vi "Main.vi"(11 "Module Number":dbl=1.0) -> ()   [LabVIEW 2015, in "Copy of Untitled Library 1.lvlib"]
uses:
  Copy of Untitled Library 1.lvlib
  Controls/Control 1.ctl
  <vilib>/Utility/miscctls.llb/LVPointTypeDef.ctl
  Controls/Enum Constant.ctl
  <userlib>/origin_lib_main/ui_msg_lib/CTRL/Display MSG Types.ctl
  <userlib>/origin_lib_main/ui_msg_lib/MSG Library.lvlib
  <userlib>/origin_lib_main/virtual_keyboard_lib/virtual_keyboard.lvlib
panel:
  out "Primery key values":string[](array[string])
  out "subarray":string[](array[string])
  in  "Tab Control":enum32{"Page 1", "Page 2"}(tab)
  in  "close button":bool
  in  "Close Batch":bool
  in  "Open Batch":bool
  in  "New Product":bool
  in  "Delete Product":bool
  in  "Reset Button":bool
  in  "Edit Button":bool
  in  "Delete Batch":bool
  in  "ADD Batch":bool
  in  "Logo 4":bool
  in  "Page Header 2":string="                                                                           BATCH PAGE"
  in  "Check Batch Status":bool caption="Open"
  in  "Batch Data 3":T1 caption="Batch Data"
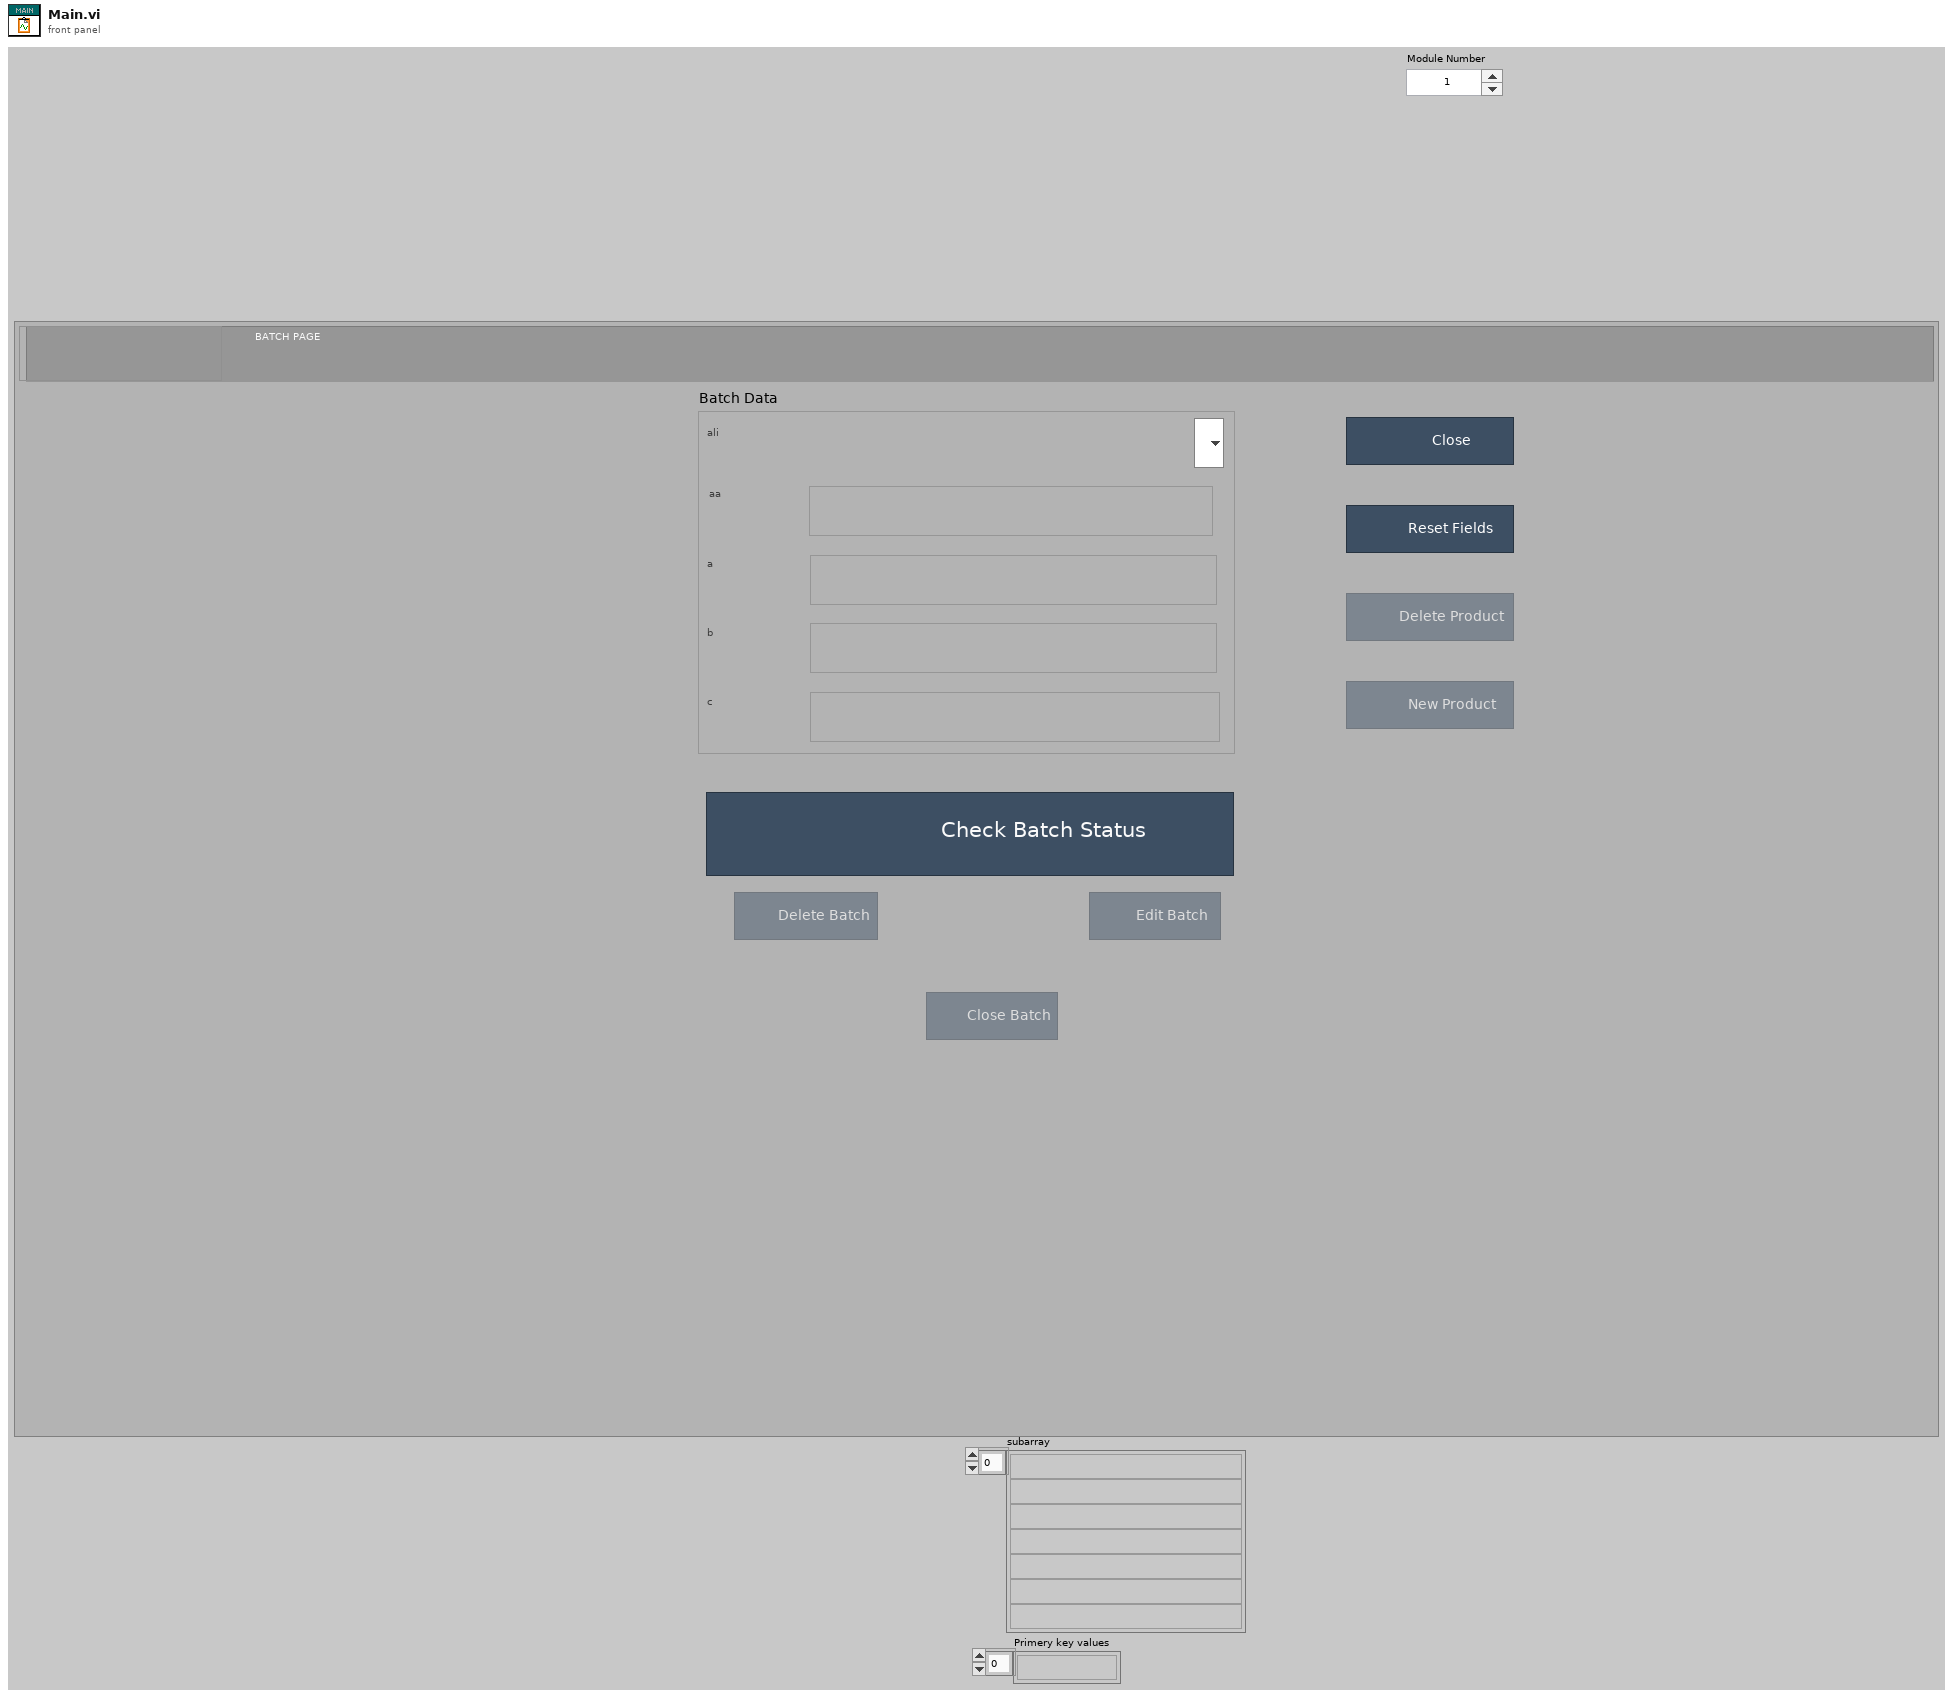
[diagram p1: front panel]
types:
  T1 = typedef "Copy of Untitled Library 1.lvlib/Control 1.ctl" = cluster{"DATA":string, "DATA 2":string, "DATA 3":string, "DATA 4":string, "DATA 5":string, "DATA 6":string, "DATA 7":string, "DATA 8":string, "DATA 9":string, "DATA 10":string, "Product":string}
  T2 = typedef "LVPointTypeDef.ctl" = cluster{"Horizontal":i16, "Vertical":i16}
  T3 = enum32{"Invalid", "Standard", "Closed", "Hidden", "Minimized", "Maximized"}
  T4 = typedef "Enum Constant.ctl" = enum16{"Init", "Read", "Write"}
  T5 = enum8{"Enabled", "Disabled", "Disabled and Grayed Out"}
  T6 = typedef "MSG Library.lvlib/Display MSG Types.ctl" = enum16{"Display MSG 1", "Display MSG 2", "Display MSG Load", "End MSG Load ", "Display 2 STR MSG"}
  T7 = typedef "FGV Data.ctl" = T8[]
  T8 = typedef "FGV Cluster Data.ctl" = cluster{"Manual/Automatic":bool, "UI Controllers ":string[], "UI Primery Key ":dbl[], "Caller Queue & MSG":T9, "Module ID":dbl, "DB Reference In":T10, "Products Columns":string[], "Cluster":cluster{"Delete Product":enum8{"Enabled", "Disabled", "Disabled and Grayed Out"}, "Add Product ":enum8{"Enabled", "Disabled", "Disabled and Grayed Out"}, "EDIT BATCH":enum8{"Enabled", "Disabled", "Disabled and Grayed Out"}, "Open Batch ":enum8{"Enabled", "Disabled", "Disabled and Grayed Out"}, "Close Batch":enum8{"Enabled", "Disabled", "Disabled and Grayed Out"}, "Delete Batch":enum8{"Enabled", "Disabled", "Disabled and Grayed Out"}, "Add Batch ":enum8{"Enabled", "Disabled", "Disabled and Grayed Out"}}}
  T9 = typedef "Queue and Caller MSG.ctl" = cluster{"Caller Queue":refnum<queue>, "Caller MSG":string}
  T10 = typedef "NI_Database_API.lvlib/Conn ObjectReference.ctl" = refnum<k1>
  T11 = cluster{"Delete Product":enum8{"Enabled", "Disabled", "Disabled and Grayed Out"}, "Add Product ":enum8{"Enabled", "Disabled", "Disabled and Grayed Out"}, "EDIT BATCH":enum8{"Enabled", "Disabled", "Disabled and Grayed Out"}, "Open Batch ":enum8{"Enabled", "Disabled", "Disabled and Grayed Out"}, "Close Batch":enum8{"Enabled", "Disabled", "Disabled and Grayed Out"}, "Delete Batch":enum8{"Enabled", "Disabled", "Disabled and Grayed Out"}, "Add Batch ":enum8{"Enabled", "Disabled", "Disabled and Grayed Out"}}
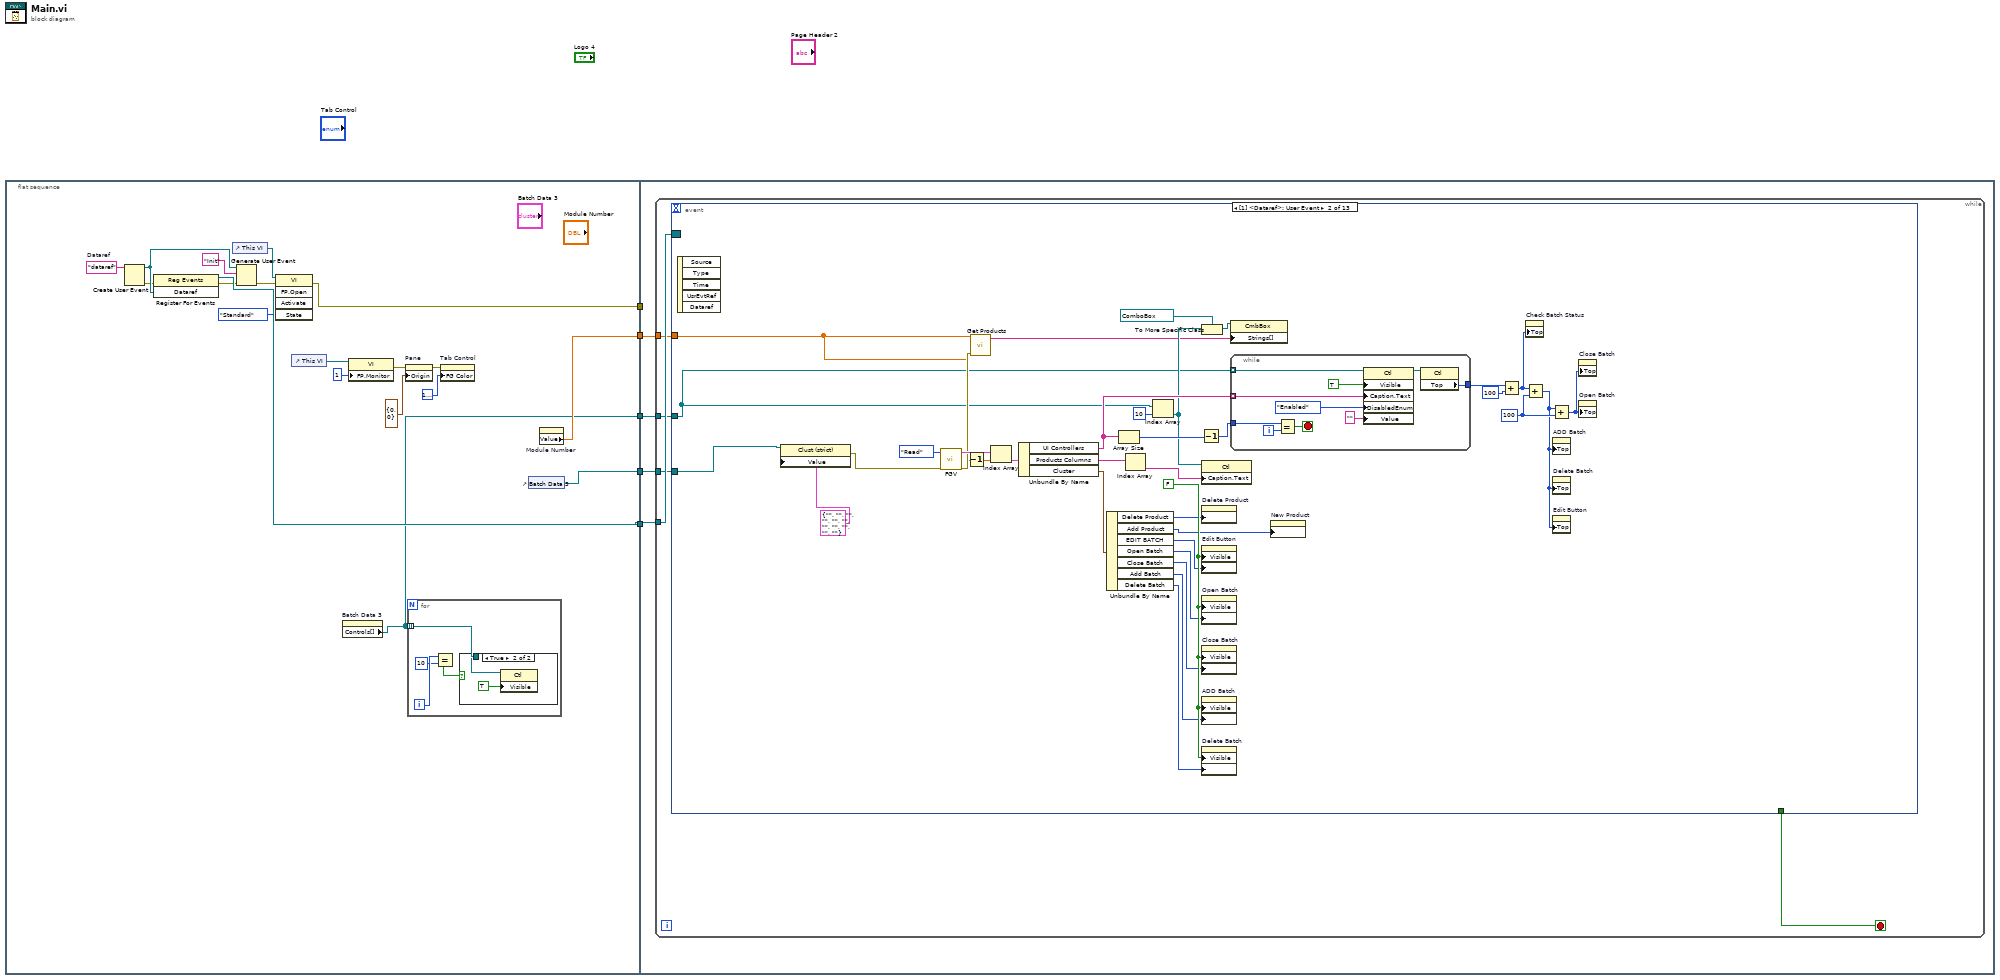
[diagram p0: block diagram]
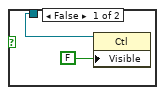
[diagram p2: hidden frame]
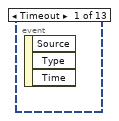
[diagram p3: hidden frame]
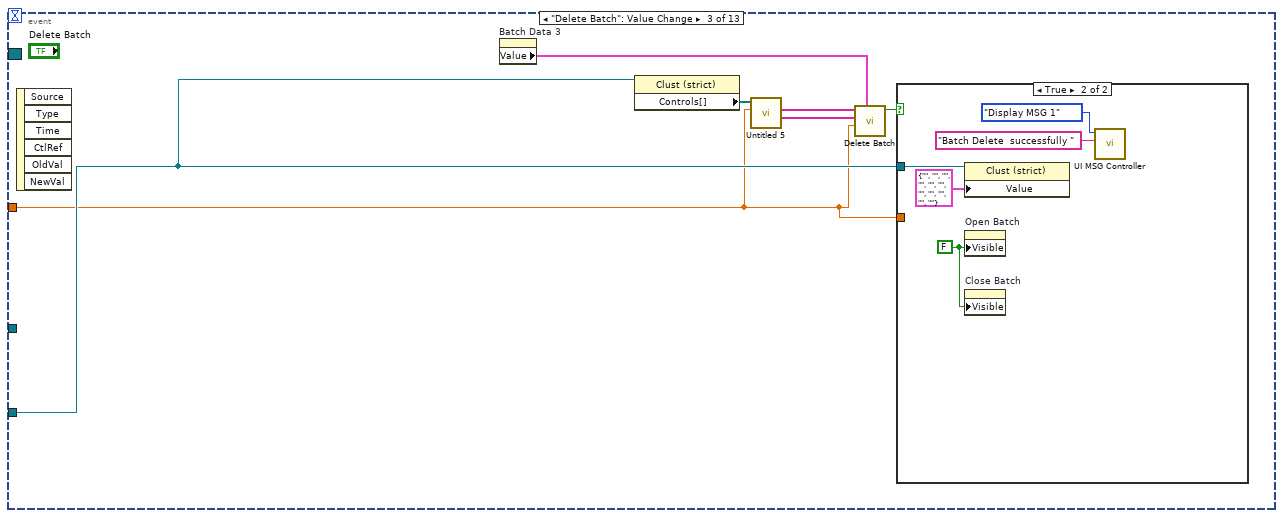
[diagram p4: hidden frame]
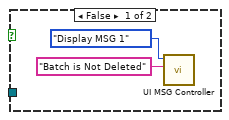
[diagram p5: hidden frame]
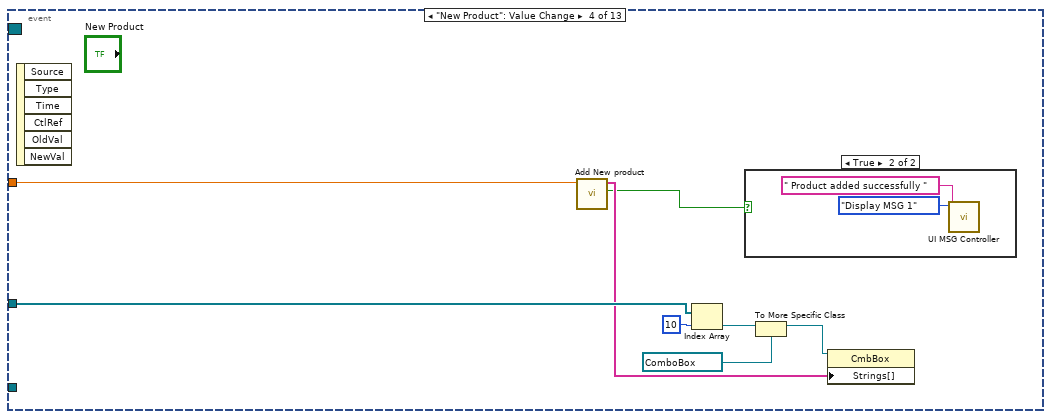
[diagram p6: hidden frame]
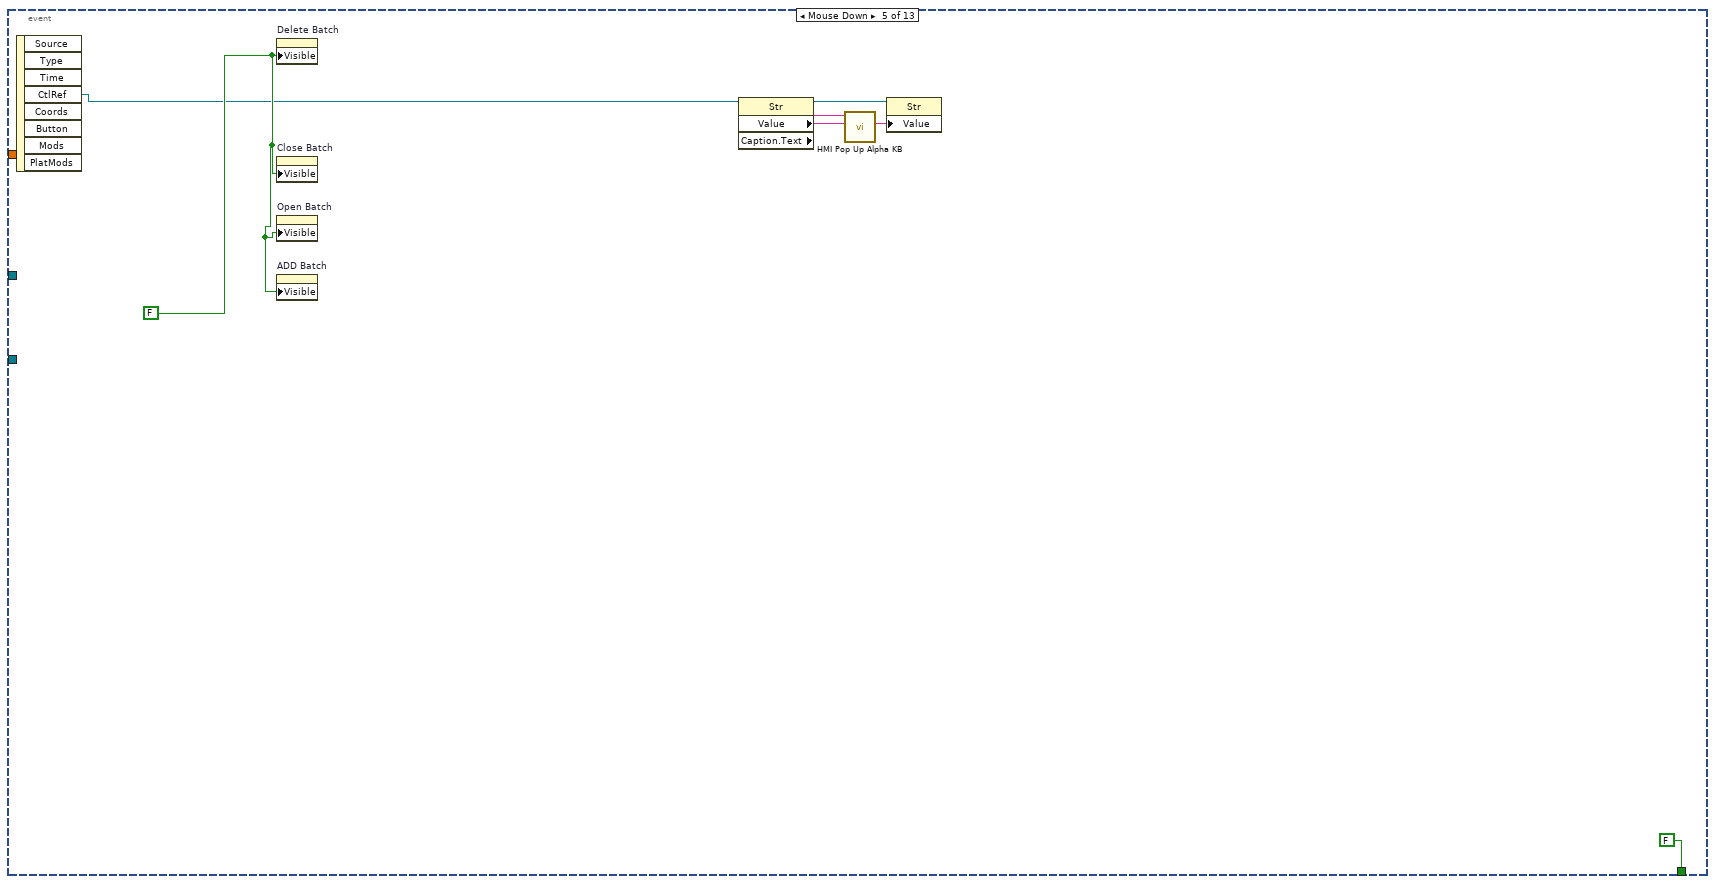
[diagram p8: hidden frame]
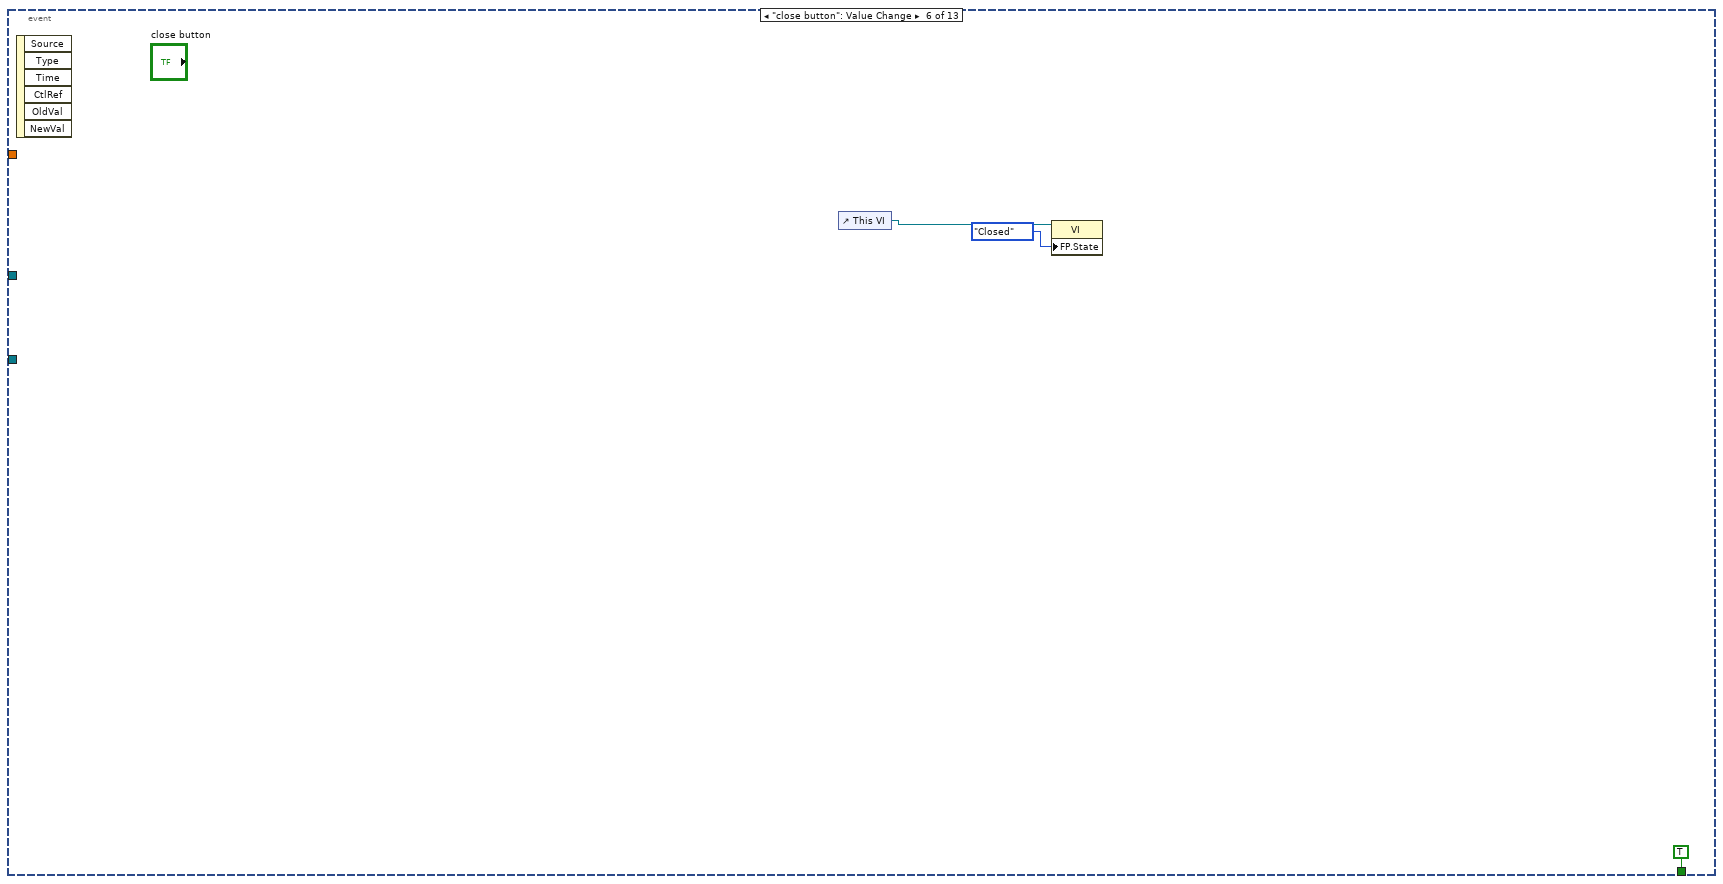
[diagram p9: hidden frame]
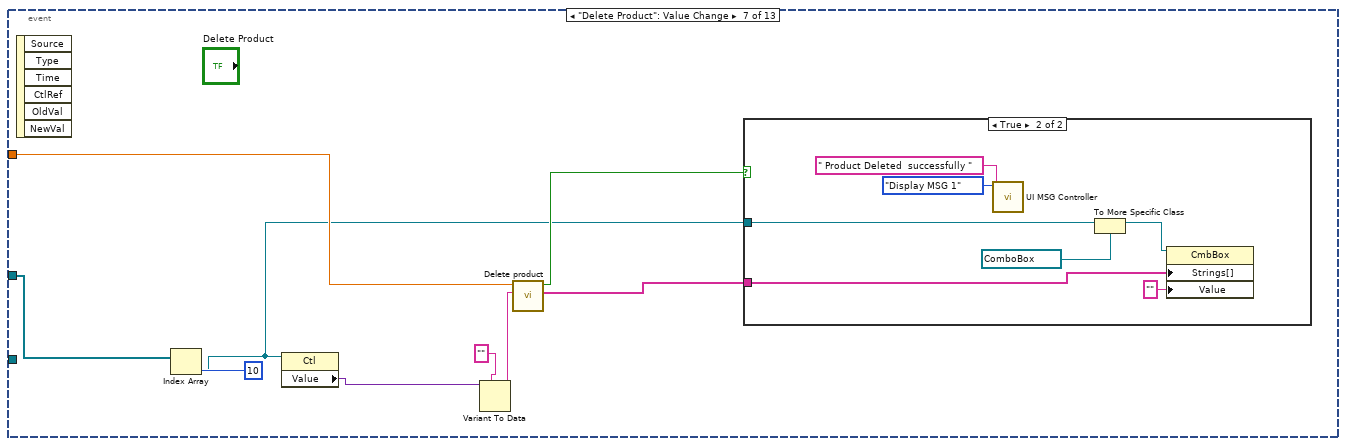
[diagram p10: hidden frame]
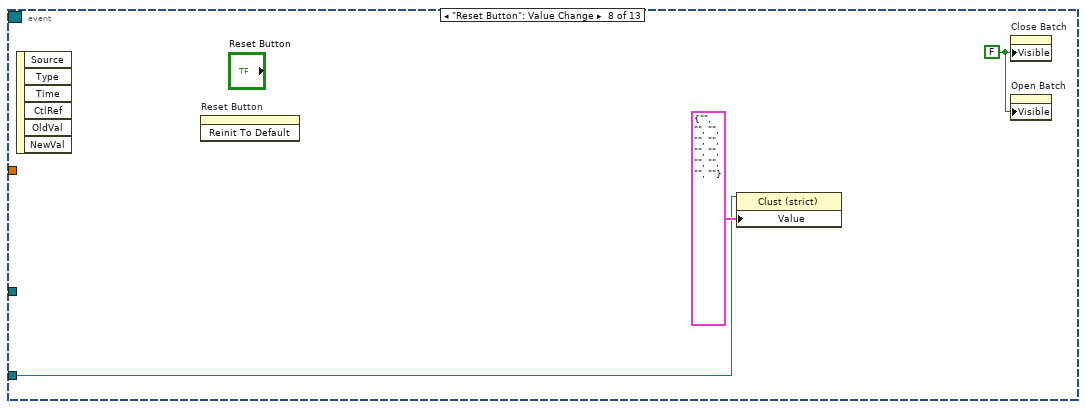
[diagram p12: hidden frame]
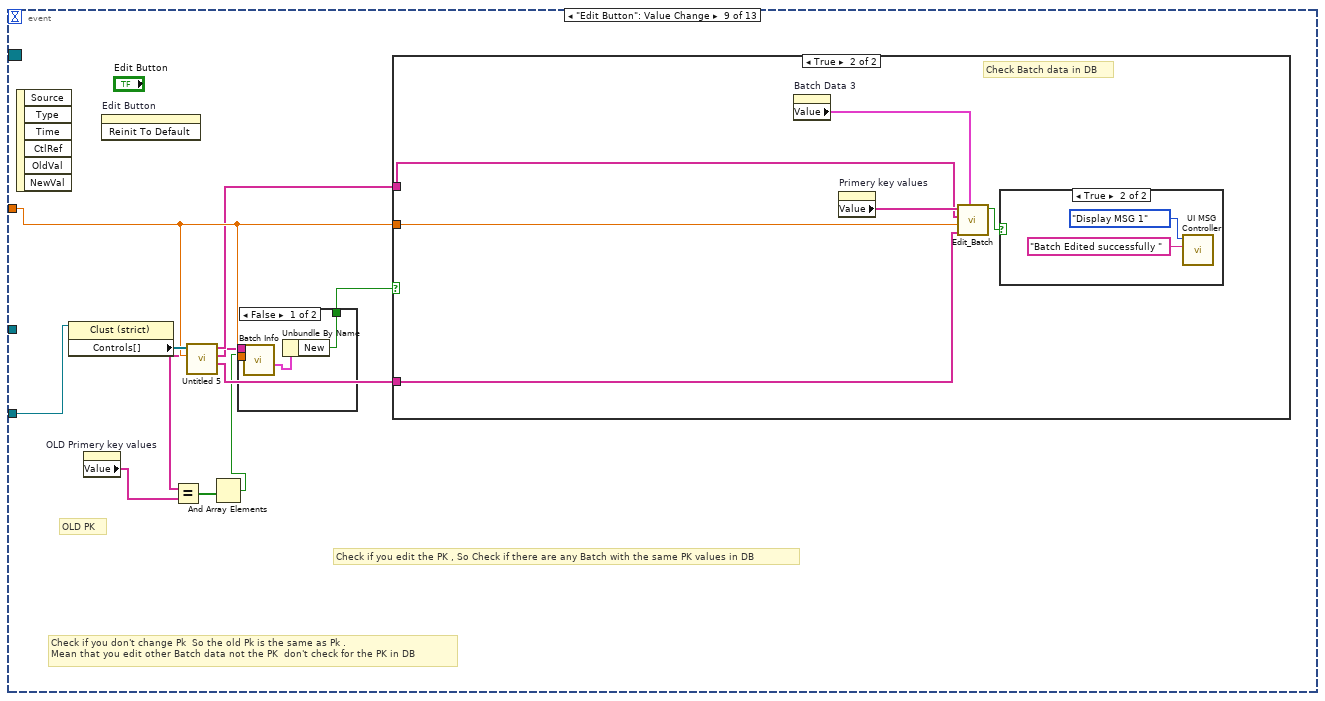
[diagram p13: hidden frame]
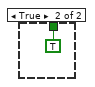
[diagram p14: hidden frame]
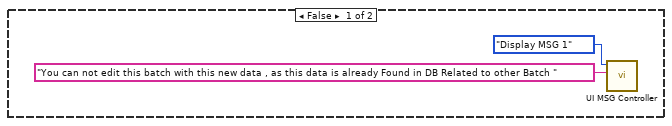
[diagram p15: hidden frame]
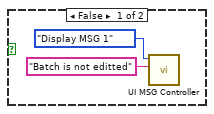
[diagram p16: hidden frame]
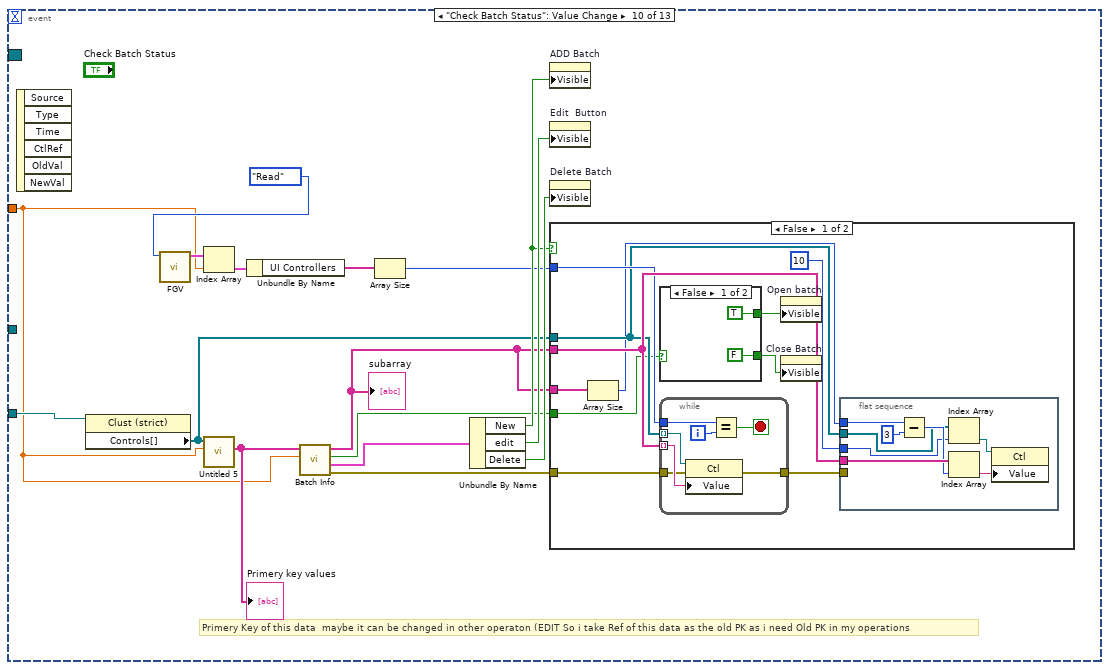
[diagram p17: hidden frame]
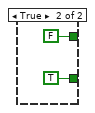
[diagram p18: hidden frame]
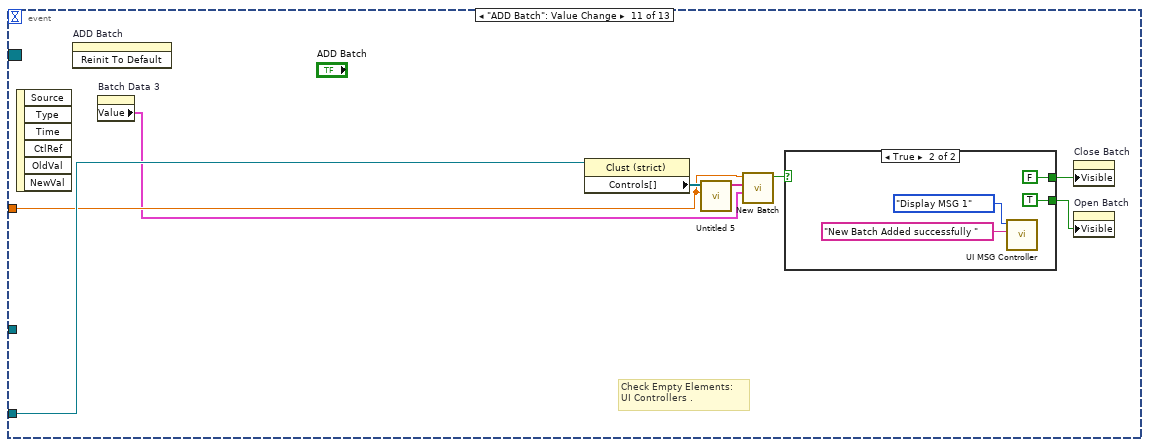
[diagram p20: hidden frame]
diagram:
  n1 = flat-sequence {
    tunnel: [w21] -> w5
    tunnel: [w15] -> w4
    tunnel: [w8] -> w3
    tunnel: [w7] -> w2
    tunnel: [w6] -> w1
    tunnel: w5 -> [w36]
    tunnel: w4 -> [_]
    tunnel: w3 -> [w35]
    tunnel: w2 -> [w34]
    tunnel: w1 -> [w33]
    frame #0 {
      w24 = "dataref"  # Dataref
      n2 = Create User Event(user event datatype=w24) -> (user event=w22:refnum<user-event>, error out=w19:errorcluster)  [unwired: 1 in]
      n3 = register-events(error in=w19, w22) -> (reference out=w21:refnum<event-registration>, error out=w20:errorcluster)  [unwired: 1 in]
      n4 = control-ref of="This VI"() -> (w18:refnum<vi>)
      n5 = Generate User Event(user event=w22, event data cluster="Init" ("event data"), error in=w20) -> (error out=w16:errorcluster)  [unwired: 1 in, 1 out]
      n6 = invoke class="VI" method="FP.Open"(reference=w18, error in=w16, "State"=T3."Standard") -> (error out=w15:errorcluster)  [unwired: 2 in, 4 out]
      n7 = control-ref of="This VI"() -> (w14:refnum<vi>)
      n8 = property on="Batch Data 3" class="Clust (strict)"() -> ("Controls[]"=w7:refnum<vi>[])  [unwired: 2 in, 2 out]
      n9 = property class="VI"(reference=w14, "FP.Monitor"=u16 1 ("Front Panel Window:Monitor")) -> (error out=w11:errorcluster)  [unwired: 1 in, 1 out]
      n10 = property on="Pane" class="Pane"(error in=w11, "Origin"=T2 {"Horizontal"=0, "Vertical"=0}) -> (error out=w9:errorcluster)  [unwired: 1 in, 1 out]
      n11 = for {
        tunnel: w7 -> [w28] mode=indexing
        i -> [w27]
        n12 = Equal?(x=w27, y=10) -> (x = y?=w25:bool)
        n13 = case shown="True" w25 {
          tunnel: w28 -> [w29 w31]
          frame False {
            n14 = property class="Ctl"(reference=w29, "Visible"=FALSE) -> ()  [unwired: 1 in, 2 out]
          }
          frame True {
            n15 = property class="Ctl"(reference=w31, "Visible"=TRUE) -> ()  [unwired: 1 in, 2 out]
          }
        }
      }
      n16 = property on="Tab Control" class="TabCtl (strict)"(error in=w9, "FG Color"=u32 16777225) -> ()  [unwired: 1 in, 2 out]
      n17 = control-ref of="Batch Data 3"() -> (w6:refnum<vi>)
      n18 = property on="Module Number" class="DigNum (strict)"() -> ("Value"=w8:dbl)  [unwired: 2 in, 2 out]
    }
    frame #1 {
      n19 = while {
        tunnel: w36 -> [w41]
        tunnel: w35 -> [w40]
        tunnel: w34 -> [w39]
        tunnel: w33 -> [w38]
        stop <- w37 stop-if-true
        n20 = event shown="[1] <Dataref>: User Event" {
          selector: w41 -> [_ _ _ _ _ _ _ _ _ _ _ _ _]
          dyn-events: _ -> [_ _ _ _ _ _ _ _ _ _ _ _ _]
          timeout: _ -> [_ _ _ _ _ _ _ _ _ _ _ _ _]
          tunnel: w40 -> [_ w50 w88 w108 _ _ w129 _ w147 w169 w214 w230 w250]
          tunnel: w39 -> [_ w52 _ w103 _ _ w128 _ _ _ _ _ _]
          tunnel: w38 -> [_ w51 w89 _ _ _ _ w137 w146 w173 w215 w229 w249]
          tunnel: [_ _ _ _ FALSE TRUE _ _ _ _ _ _ _] -> w37
          event Timeout {
            n21 = event-data() -> ()  [unwired: 1 in, 3 out]
          }
          event User Event {
            w66 = 100 ("y")
            w67 = FALSE ("Visible")
            n22 = event-data() -> ()  [unwired: 1 in, 5 out]
            n23 = property class="Clust (strict)"(reference=w51, "Value"=T1 {"DATA"="", "DATA 2"="", "DATA 3"="", "DATA 4"="", "DATA 5"="", "DATA 6"="", "DATA 7"="", "DATA 8"="", "DATA 9"="", "DATA 10"="", "Product"=""}) -> (error out=w53:errorcluster)  [unwired: 1 in, 1 out]
            n24 = call "FGV.vi"("error out 2"=w53, "Enum"=Enum_Constant."Read") -> ("error out"=w60:errorcluster, "Read Data"=w75:T7)  [unwired: 8 in]
            n25 = Decrement(x=w50) -> (x-1=w55:dbl)
            n26 = call "Get Products.vi"("error in (no error) 5"=w60, "Module Number  2"=w50) -> ("subarray"=w56:string[])  [unwired: 8 in, 1 out]
            n27 = Index Array(array=w75, index=w55) -> (element=w74:T8)
            n28 = Unbundle By Name(w74) -> ("UI Controllers"=w73:string[], "Products Columns"=w62:string[], "Cluster"=w49:T11)
            n29 = Unbundle By Name(w49) -> ("Delete Product"=w48:T5, "Add Product"=w47:T5, "EDIT BATCH"=w46:T5, "Open Batch"=w45:T5, "Close Batch"=w44:T5, "Add Batch"=w43:T5, "Delete Batch"=w42:T5)
            n30 = Array Size(array=w73) -> (size(s)=w70:i32)
            n31 = Index Array(array=w62) -> (element=w61:string)  [unwired: 1 in]
            n32 = Index Array(array=w52, index=10) -> (element=w57:refnum<vi>)
            n33 = Decrement(x=w70) -> (x-1=w69:i32)
            n34 = To More Specific Class(target class=refnum<vi> refnum ("Product"), reference=w57) -> (specific class reference=w59:refnum<vi>)  [unwired: 1 in, 1 out]
            n35 = property class="Ctl"(reference=w57, "Caption.Text"=w61) -> ()  [unwired: 1 in, 2 out]
            n36 = property on="Delete Product" class="Bool"("DisabledEnum"=w48) -> ()  [unwired: 2 in, 2 out]
            n37 = property on="Edit Button" class="Bool"("Visible"=w67, "DisabledEnum"=w46) -> ()  [unwired: 2 in, 2 out]
            n38 = property on="Open Batch" class="Bool"("Visible"=w67, "DisabledEnum"=w45) -> ()  [unwired: 2 in, 2 out]
            n39 = property on="Close Batch" class="Bool"("Visible"=w67, "DisabledEnum"=w44) -> ()  [unwired: 2 in, 2 out]
            n40 = property on="ADD Batch" class="Bool (strict)"("Visible"=w67, "DisabledEnum"=w43) -> ()  [unwired: 2 in, 2 out]
            n41 = property on="Delete Batch" class="Bool"("Visible"=w67, "DisabledEnum"=w42) -> ()  [unwired: 2 in, 2 out]
            n42 = property class="CmbBox"(reference=w59, "Strings[]"=w56) -> ()  [unwired: 1 in, 2 out]
            n43 = while {
              tunnel: w73 -> [w82] mode=indexing
              tunnel: w69 -> [w86]
              tunnel: [w80] -> w71
              tunnel: w52 -> [w79] mode=indexing
              i -> [w85]
              stop <- w84 stop-if-true
              n44 = Equal?(x=w86, y=w85) -> (x = y?=w84:bool)
              n45 = property class="Ctl"(reference=w79, "Visible"=TRUE, "Caption.Text"=w82, "DisabledEnum"=T5."Enabled" ("Disabled"), "Value"="" ("String")) -> (reference out=w81:refnum<vi>)  [unwired: 1 in, 1 out]
              n46 = property class="Ctl"(reference=w81) -> ("Top"=w80:i32)  [unwired: 1 in, 2 out]
            }
            n47 = property on="New Product" class="Bool"("DisabledEnum"=w47) -> ()  [unwired: 2 in, 2 out]
            n48 = Add(x=w71, y=100) -> (x+y=w68:i32)
            n49 = Add(x=w68, y=w66) -> (x+y=w65:i32)
            n50 = property on="Check Batch Status" class="Bool"("Top"=w68) -> ()  [unwired: 2 in, 2 out]
            n51 = Add(x=w65, y=w66) -> (x+y=w64:i32)
            n52 = property on="ADD Batch" class="Bool (strict)"("Top"=w65) -> ()  [unwired: 2 in, 2 out]
            n53 = property on="Delete Batch" class="Bool"("Top"=w65) -> ()  [unwired: 2 in, 2 out]
            n54 = property on="Edit Button" class="Bool"("Top"=w65) -> ()  [unwired: 2 in, 2 out]
            n55 = property on="Close Batch" class="Bool"("Top"=w64) -> ()  [unwired: 2 in, 2 out]
            n56 = property on="Open Batch" class="Bool"("Top"=w64) -> ()  [unwired: 2 in, 2 out]
          }
          event "Delete Batch": Value Change {
            n57 = event-data() -> ()  [unwired: 1 in, 6 out]
            n58 = property on="Batch Data 3" class="Clust (strict)"() -> ("Value"=w87:T1)  [unwired: 2 in, 2 out]
            n59 = property class="Clust (strict)"(reference=w89) -> ("Controls[]"=w93:refnum<vi>[])  [unwired: 1 in, 2 out]
            n60 = call "Untitled 5.vi"("Module Number"=w88, "Controls[]"=w93) -> ("Primery key Names"=w91:string[], "Primery key values"=w92:string[])  [unwired: 7 in, 1 out]
            n61 = call "Delete Batch .vi"("Batch Data 3"=w87, "Module Number"=w88, "Primery key names"=w91, "Primery key last values"=w92) -> ("Sucess ?"=w90:bool)  [unwired: 7 in]
            n62 = case shown="True" w90 {
              tunnel: w89 -> [_ w98]
              tunnel: w88 -> [_ _]
              frame False {
                n63 = call <userlib>:"UI MSG Controller.vi"("MSG"="Batch is Not Deleted", "Display MSG Type"=Display_MSG_Types."Display MSG 1") -> ()  [unwired: 6 in, 4 out]
              }
              frame True {
                w96 = FALSE ("Visible")
                n64 = property class="Clust (strict)"(reference=w98, "Value"=T1 {"DATA"="", "DATA 2"="", "DATA 3"="", "DATA 4"="", "DATA 5"="", "DATA 6"="", "DATA 7"="", "DATA 8"="", "DATA 9"="", "DATA 10"="", "Product"=""}) -> ()  [unwired: 1 in, 2 out]
                n65 = property on="Open Batch" class="Bool"("Visible"=w96) -> ()  [unwired: 2 in, 2 out]
                n66 = property on="Close Batch" class="Bool"("Visible"=w96) -> ()  [unwired: 2 in, 2 out]
                n67 = call <userlib>:"UI MSG Controller.vi"("MSG"="Batch Delete  successfully ", "Display MSG Type"=Display_MSG_Types."Display MSG 1") -> ()  [unwired: 6 in, 4 out]
              }
            }
          }
          event "New Product": Value Change {
            n68 = event-data() -> ()  [unwired: 1 in, 6 out]
            n69 = call "Add New product.vi"("Module Number  2"=w108) -> ("Sucess ?"=w101:bool, "subarray"=w102:string[])  [unwired: 8 in, 1 out]
            n70 = Index Array(array=w103, index=10) -> (element=w104:refnum<vi>)
            n71 = case shown="True" w101 {
              frame False {
              }
              frame True {
                n72 = call <userlib>:"UI MSG Controller.vi"("MSG"=" Product added successfully ", "Display MSG Type"=Display_MSG_Types."Display MSG 1") -> ()  [unwired: 6 in, 4 out]
              }
            }
            n73 = To More Specific Class(target class=refnum<vi> refnum ("Product"), reference=w104) -> (specific class reference=w106:refnum<vi>)  [unwired: 1 in, 1 out]
            n74 = property class="CmbBox"(reference=w106, "Strings[]"=w102) -> ()  [unwired: 1 in, 2 out]
          }
          event Mouse Down {
            w117 = FALSE ("Visible")
            n75 = event-data() -> ("CtlRef"=w112:refnum<vi>)  [unwired: 1 in, 7 out]
            n76 = property on="Delete Batch" class="Bool"("Visible"=w117) -> ()  [unwired: 2 in, 2 out]
            n77 = property on="Close Batch" class="Bool"("Visible"=w117) -> ()  [unwired: 2 in, 2 out]
            n78 = property on="Open Batch" class="Bool"("Visible"=w117) -> ()  [unwired: 2 in, 2 out]
            n79 = property on="ADD Batch" class="Bool (strict)"("Visible"=w117) -> ()  [unwired: 2 in, 2 out]
            n80 = property class="Str"(reference=w112) -> (reference out=w114:refnum<vi>, "Value"=w116:string, "Caption.Text"=w113:string)  [unwired: 1 in, 1 out]
            n81 = call <userlib>:"HMI Pop Up Alpha KB.vi"("String In"=w116, "Message In"=w113) -> ("String Out"=w115:string)  [unwired: 7 in, 2 out]
            n82 = property class="Str"(reference=w114, "Value"=w115) -> ()  [unwired: 1 in, 2 out]
          }
          event "close button": Value Change {
            n83 = event-data() -> ()  [unwired: 1 in, 6 out]
            n84 = control-ref of="This VI"() -> (w120:refnum<vi>)
            n85 = property class="VI"(reference=w120, "FP.State"=T3."Closed" ("Front Panel Window:State")) -> ()  [unwired: 1 in, 2 out]
          }
          event "Delete Product": Value Change {
            n86 = event-data() -> ()  [unwired: 1 in, 6 out]
            n87 = Index Array(array=w128, index=10) -> (element=w121:refnum<vi>)
            n88 = property class="Ctl"(reference=w121) -> ("Value"=w126:variant)  [unwired: 1 in, 2 out]
            n89 = Variant To Data(type="", Variant=w126) -> (data=w124:string)  [unwired: 1 in, 1 out]
            n90 = call "Delete product.vi"("String"=w124, "Module Number  2"=w129) -> ("subarray"=w122:string[], "Sucess ?"=w123:bool)  [unwired: 7 in, 1 out]
            n91 = case shown="True" w123 {
              tunnel: w122 -> [_ w132]
              tunnel: w121 -> [_ w131]
              frame False {
              }
              frame True {
                n92 = call <userlib>:"UI MSG Controller.vi"("MSG"=" Product Deleted  successfully ", "Display MSG Type"=Display_MSG_Types."Display MSG 1") -> ()  [unwired: 6 in, 4 out]
                n93 = To More Specific Class(target class=refnum<vi> refnum ("Product"), reference=w131) -> (specific class reference=w133:refnum<vi>)  [unwired: 1 in, 1 out]
                n94 = property class="CmbBox"(reference=w133, "Strings[]"=w132, "Value"="") -> ()  [unwired: 1 in, 2 out]
              }
            }
          }
          event "Reset Button": Value Change {
            w138 = FALSE ("Visible")
            n95 = event-data() -> ()  [unwired: 1 in, 6 out]
            n96 = invoke on="Reset Button" class="Bool" method="Reinit To Default"() -> ()  [unwired: 3 in, 3 out]
            n97 = property class="Clust (strict)"(reference=w137, "Value"=T1 {"DATA"="", "DATA 2"="", "DATA 3"="", "DATA 4"="", "DATA 5"="", "DATA 6"="", "DATA 7"="", "DATA 8"="", "DATA 9"="", "DATA 10"="", "Product"=""}) -> ()  [unwired: 1 in, 2 out]
            n98 = property on="Close Batch" class="Bool"("Visible"=w138) -> ()  [unwired: 2 in, 2 out]
            n99 = property on="Open Batch" class="Bool"("Visible"=w138) -> ()  [unwired: 2 in, 2 out]
          }
          event "Edit Button": Value Change {
            # "Check if you don't change Pk  So the old Pk is the same as Pk .\nMean that you edit other Batch data not the PK  don't check for the PK in DB"
            # "Check if you edit the PK , So Check if there are any Batch with the same PK values in DB"
            # "OLD PK"
            n100 = event-data() -> ()  [unwired: 1 in, 6 out]
            n101 = property class="Clust (strict)"(reference=w146) -> ("Controls[]"=w148:refnum<vi>[])  [unwired: 1 in, 2 out]
            n102 = property on="OLD Primery key values" class="Arr (strict)"() -> ("Value"=w142:string[])  [unwired: 2 in, 2 out]
            n103 = invoke on="Edit Button" class="Bool" method="Reinit To Default"() -> ()  [unwired: 3 in, 3 out]
            n104 = call "Untitled 5.vi"("Module Number"=w147, "Controls[]"=w148) -> ("Primery key Names"=w144:string[], "Primery key values"=w143:string[], "BatchData"=w145:string[])  [unwired: 7 in]
            n105 = Equal?(x=w143, y=w142) -> (x = y?=w141:bool[])
            n106 = And Array Elements(Boolean array=w141) -> (logical AND=w140:bool)
            n107 = case shown="False" w140 {
              tunnel: [w152 TRUE ("New")] -> w149
              tunnel: w147 -> [w151 _]
              tunnel: w143 -> [w150 _]
              frame False {
                n108 = call "Batch Info.vi"("Module Number  2"=w151, "Array"=w150) -> ("Cluster"=w153:cluster{"New":bool, "edit":bool, "Delete":bool})  [unwired: 6 in, 3 out]
                n109 = Unbundle By Name(w153) -> ("New"=w152:bool)
              }
              frame True {
              }
            }
            n110 = case shown="True" w149 {
              tunnel: w147 -> [_ w160]
              tunnel: w145 -> [_ w158]
              tunnel: w144 -> [_ w157]
              frame False {
                n111 = call <userlib>:"UI MSG Controller.vi"("MSG"="You can not edit this batch with this new data , as this data is already Found in DB Related to other Batch ", "Display MSG Type"=Display_MSG_Types."Display MSG 1") -> ()  [unwired: 6 in, 4 out]
              }
              frame True {
                # "Check Batch data in DB"
                n112 = property on="Batch Data 3" class="Clust (strict)"() -> ("Value"=w159:T1)  [unwired: 2 in, 2 out]
                n113 = property on="Primery key values" class="Arr (strict)"() -> ("Value"=w162:string[])  [unwired: 2 in, 2 out]
                n114 = call "Edit_Batch.vi"("Batch Data 3"=w159, "Primery key names"=w157, "Module Number  3"=w160, "Batch data"=w158, "Primery key last values"=w162) -> ("Sucess ?"=w161:bool)  [unwired: 5 in, 1 out]
                n115 = case shown="True" w161 {
                  frame False {
                    n116 = call <userlib>:"UI MSG Controller.vi"("MSG"="Batch is not editted", "Display MSG Type"=Display_MSG_Types."Display MSG 1") -> ()  [unwired: 6 in, 4 out]
                  }
                  frame True {
                    n117 = call <userlib>:"UI MSG Controller.vi"("MSG"="Batch Edited successfully ", "Display MSG Type"=Display_MSG_Types."Display MSG 1") -> ()  [unwired: 6 in, 4 out]
                  }
                }
              }
            }
          }
          event "Check Batch Status": Value Change {
            # "Primery Key of this data  maybe it can be changed in other operaton (EDIT So i take Ref of this data as the old PK as i need Old PK in my operations"
            n118 = event-data() -> ()  [unwired: 1 in, 6 out]
            n119 = property class="Clust (strict)"(reference=w173) -> ("Controls[]"=w176:refnum<vi>[])  [unwired: 1 in, 2 out]
            n120 = call "FGV.vi"("Enum"=Enum_Constant."Read") -> ("Read Data"=w171:T7)  [unwired: 9 in, 1 out]
            n121 = Index Array(array=w171, index=w169) -> (element=w170:T8)
            n122 = call "Untitled 5.vi"("Module Number"=w169, "Controls[]"=w176) -> ("Primery key values"=w177:string[])  [unwired: 7 in, 2 out]
            "Primery key values" <- w177
            n123 = Unbundle By Name(w170) -> ("UI Controllers"=w168:string[])
            n124 = call "Batch Info.vi"("Module Number  2"=w169, "Array"=w177) -> ("error out"=w175:errorcluster, "Cluster"=w182:cluster{"New":bool, "edit":bool, "Delete":bool}, "Batch Open or Not"=w174:bool, "subarray"=w167:string[])  [unwired: 6 in]
            "subarray" <- w167
            n125 = Array Size(array=w168) -> (size(s)=w178:i32)
            n126 = Unbundle By Name(w182) -> ("New"=w179:bool, "edit"=w181:bool, "Delete"=w180:bool)
            n127 = property on="ADD Batch" class="Bool (strict)"("Visible"=w179) -> ()  [unwired: 2 in, 2 out]
            n128 = property on="Edit  Button" class="Bool"("Visible"=w181) -> ()  [unwired: 2 in, 2 out]
            n129 = property on="Delete Batch" class="Bool"("Visible"=w180) -> ()  [unwired: 2 in, 2 out]
            n130 = case shown="False" w179 {
              tunnel: w167 -> [w193 _]
              tunnel: w178 -> [w192 _]
              tunnel: w176 -> [w191 _]
              tunnel: w175 -> [w189 _]
              tunnel: w174 -> [w187 _]
              tunnel: w167 -> [w184 _]
              frame False {
                n131 = Array Size(array=w184) -> (size(s)=w183:i32)
                n132 = case shown="False" w187 {
                  tunnel: [FALSE ("Visible") TRUE ("Visible")] -> w186
                  tunnel: [TRUE ("Visible") FALSE ("Visible")] -> w185
                  frame False {
                  }
                  frame True {
                  }
                }
                n133 = while {
                  tunnel: w191 -> [w210] mode=indexing
                  tunnel: w193 -> [w209] mode=indexing
                  tunnel: w192 -> [w208]
                  tunnel: w189 -> [w207]
                  tunnel: [w206] -> w188
                  i -> [w212]
                  stop <- w211 stop-if-true
                  n134 = property class="Ctl"(reference=w210, error in=w207, "Value"=w209) -> (error out=w206:errorcluster)  [unwired: 1 out]
                  n135 = Equal?(x=w208, y=w212) -> (x = y?=w211:bool)
                }
                n136 = property on="Open batch" class="Bool"("Visible"=w185) -> ()  [unwired: 2 in, 2 out]
                n137 = property on="Close Batch" class="Bool"("Visible"=w186) -> ()  [unwired: 2 in, 2 out]
                n138 = flat-sequence {
                  tunnel: w193 -> [w205]
                  tunnel: w183 -> [w203]
                  tunnel: w191 -> [w200]
                  tunnel: 10 ("index") -> [w199]
                  tunnel: w188 -> [_]
                  frame #0 {
                    n139 = Subtract(x=w203, y=3) -> (x-y=w201:i32)
                    n140 = Index Array(array=w200, index=w199) -> (element=w198:refnum<vi>)
                    n141 = Index Array(array=w205, index=w201) -> (element=w204:string)
                    n142 = property class="Ctl"(reference=w198, "Value"=w204) -> ()  [unwired: 1 in, 2 out]
                  }
                }
              }
              frame True {
              }
            }
          }
          event "ADD Batch": Value Change {
            # "Check Empty Elements: \nUI Controllers ."
            n143 = event-data() -> ()  [unwired: 1 in, 6 out]
            n144 = invoke on="ADD Batch" class="Bool (strict)" method="Reinit To Default"() -> ()  [unwired: 3 in, 3 out]
            n145 = property on="Batch Data 3" class="Clust (strict)"() -> ("Value"=w213:T1)  [unwired: 2 in, 2 out]
            n146 = property class="Clust (strict)"(reference=w215) -> ("Controls[]"=w220:refnum<vi>[])  [unwired: 1 in, 2 out]
            n147 = call "Untitled 5.vi"("Module Number"=w214, "Controls[]"=w220) -> ("BatchData"=w219:string[])  [unwired: 7 in, 2 out]
            n148 = call "New Batch.vi"("Batch Data 3"=w213, "Batch data"=w219, "Module Number  3"=w214) -> ("Sucess ?"=w218:bool)  [unwired: 7 in, 1 out]
            n149 = case shown="True" w218 {
              tunnel: [w221 TRUE ("Visible")] -> w217
              tunnel: [w221 FALSE ("Visible")] -> w216
              frame False {
                w221 = FALSE ("Visible")
                n150 = call <userlib>:"UI MSG Controller.vi"("MSG"="New Batch is Not added", "Display MSG Type"=Display_MSG_Types."Display MSG 1") -> ()  [unwired: 6 in, 4 out]
              }
              frame True {
                n151 = call <userlib>:"UI MSG Controller.vi"("MSG"="New Batch Added successfully ", "Display MSG Type"=Display_MSG_Types."Display MSG 1") -> ()  [unwired: 6 in, 4 out]
              }
            }
            n152 = property on="Close Batch" class="Bool"("Visible"=w216) -> ()  [unwired: 2 in, 2 out]
            n153 = property on="Open Batch" class="Bool"("Visible"=w217) -> ()  [unwired: 2 in, 2 out]
          }
          event "Open Batch": Value Change {
            n154 = event-data() -> ()  [unwired: 1 in, 6 out]
            n155 = property on="Batch Data 3" class="Clust (strict)"() -> ("Value"=w228:T1)  [unwired: 2 in, 2 out]
            n156 = property class="Clust (strict)"(reference=w229) -> ("Controls[]"=w231:refnum<vi>[])  [unwired: 1 in, 2 out]
            n157 = property on="Primery key values" class="Arr (strict)"() -> ("Value"=w233:string[])  [unwired: 2 in, 2 out]
            n158 = call "Check open batches .vi"("Module Number  2"=w230) -> ("Open New Batch"=w234:bool)  [unwired: 8 in, 1 out]
            n159 = call "Untitled 5.vi"("Module Number"=w230, "Controls[]"=w231) -> ("Primery key Names"=w232:string[])  [unwired: 7 in, 2 out]
            n160 = invoke on="Open Batch" class="Bool" method="Reinit To Default"() -> ()  [unwired: 3 in, 3 out]
            n161 = case shown="True" w234 {
              tunnel: w230 -> [_ w247]
              tunnel: w233 -> [_ w237]
              tunnel: w232 -> [_ w236]
              tunnel: w228 -> [_ w235]
              frame False {
              }
              frame True {
                n162 = call "Open Batch.vi"("Batch Data 3"=w235, "Primery key names"=w236, "Primery key last values"=w237, "Module Number  2"=w247) -> ("Sucess ?"=w242:bool)  [unwired: 6 in, 1 out]
                n163 = Select(t=FALSE ("Visible"), s=w242, f=TRUE ("Visible")) -> (s? t:f=w241:bool)
                n164 = Select(t=TRUE ("Visible"), s=w242, f=FALSE ("Visible")) -> (s? t:f=w240:bool)
                n165 = property on="Open batch" class="Bool"("Visible"=w241) -> ()  [unwired: 2 in, 2 out]
                n166 = property on="Close Batch" class="Bool"("Visible"=w240) -> ()  [unwired: 2 in, 2 out]
                n167 = call <userlib>:"UI MSG Controller.vi"("MSG"="Batch Opened successfully ", "Display MSG Type"=Display_MSG_Types."Display MSG 1") -> ()  [unwired: 6 in, 4 out]
              }
            }
          }
          event "Close Batch": Value Change {
            n168 = event-data() -> ()  [unwired: 1 in, 6 out]
            n169 = property on="Batch Data 3" class="Clust (strict)"() -> ("Value"=w248:T1)  [unwired: 2 in, 2 out]
            n170 = property class="Clust (strict)"(reference=w249) -> ("Controls[]"=w256:refnum<vi>[])  [unwired: 1 in, 2 out]
            n171 = property on="Primery key values" class="Arr (strict)"() -> ("Value"=w258:string[])  [unwired: 2 in, 2 out]
            n172 = call "Untitled 5.vi"("Module Number"=w250, "Controls[]"=w256) -> ("Primery key Names"=w257:string[])  [unwired: 7 in, 2 out]
            n173 = call "Close Batch.vi"("Batch Data 3"=w248, "Primery key names"=w257, "Primery key last values"=w258, "Module Number  2"=w250) -> ("Sucess ?"=w254:bool)  [unwired: 6 in, 1 out]
            n174 = Select(t="Batch Closed  successfully " ("MSG"), s=w254, f="Batch is not Closed " ("MSG")) -> (s? t:f=w251:string)
            n175 = Select(t=TRUE ("Visible"), s=w254, f=FALSE ("Visible")) -> (s? t:f=w260:bool)
            n176 = Select(t=FALSE ("Visible"), s=w254, f=TRUE ("Visible")) -> (s? t:f=w259:bool)
            n177 = property on="Open batch" class="Bool"("Visible"=w260) -> ()  [unwired: 2 in, 2 out]
            n178 = property on="Close Batch" class="Bool"("Visible"=w259) -> ()  [unwired: 2 in, 2 out]
            n179 = call <userlib>:"UI MSG Controller.vi"("MSG"=w251, "Display MSG Type"=Display_MSG_Types."Display MSG 1") -> ()  [unwired: 6 in, 4 out]
          }
        }
      }
    }
  }
